vi "RT MainSam.vi"   [LabVIEW 2014]
uses:
  controls/UI DataSam.ctl
  <vilib>/RTwatchdog.llb/Watchdog expiration actions.ctl
  <vilib>/nisyscfg/nisyscfg.lvlib
types:
  T1 = typedef "UI DataSam.ctl" = cluster{"Message":string, "Data":variant}
  T2 = typedef "Watchdog expiration actions.ctl" = cluster{"reset":bool, "occurrence":bool, "trigger protocol":enum16{"active high", "active low", "open collector"}, "trigger line":enum16{"none", "line 0", "line 1", "line 2", "line 3", "line 4", "line 5", "line 6", "line 7", "SMB line 0"}, "disable watchdog on VI exit":bool}
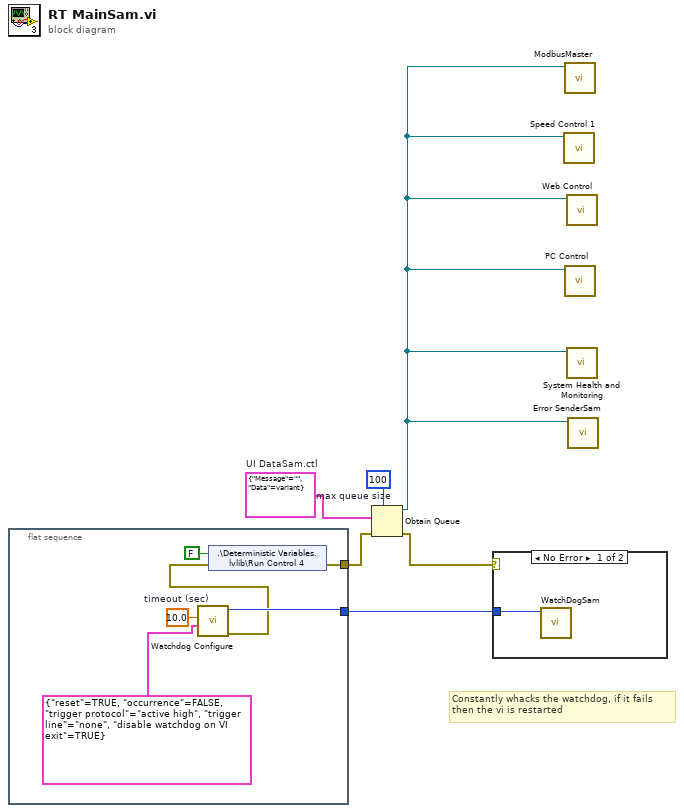
[diagram p0: block diagram]
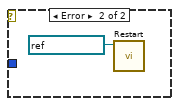
[diagram p2: hidden frame]
diagram:
  w5 = T1 {"Message"="", "Data"=variant}  # UI DataSam.ctl
  w6 = 100  # max queue size
  # "Constantly whacks the watchdog, if it fails\nthen the vi is restarted"
  n1 = flat-sequence {
    tunnel: [w12] -> w4
    tunnel: [w11] -> w2
    frame #0 {
      w9 = 10.0  # timeout (sec)
      n2 = call <vilib>:"Watchdog Configure.vi"("expiration actions"=T2 {"reset"=TRUE, "occurrence"=FALSE, "trigger protocol"=enum."active high", "trigger line"=enum."none", "disable watchdog on VI exit"=TRUE}, "timeout (1 sec)"=w9) -> ("error out"=w10:errorcluster, "watchdogID"=w11:u64)  [unwired: 2 in, 2 out]
      n3 = shared-variable ".\\Deterministic Variables.lvlib\\Run Control 4"(FALSE ("Run Control"), error in=w10) -> (error out=w12:errorcluster)
    }
  }
  n4 = Obtain Queue(max queue size (-1, unlimited)=w6, element data type=w5, error in (no error)=w4) -> (queue out=w1:refnum<queue>, error out=w3:errorcluster)  [unwired: 2 in, 1 out]
  n5 = case shown="No Error" w3 {
    tunnel: w2 -> [w13 _]
    frame No Error {
      n6 = call "WatchDogSam.vi"("watchdogID"=w13) -> ()  [unwired: 11 in]
    }
    frame Error {
      n7 = call <vilib>:"Restart.vi"("Session in"=refnum<k21> "localhost") -> ()  [unwired: 8 in, 3 out]
    }
  }
  n8 = call "Speed Control 1.vi"("queue in"=w1) -> ()  [unwired: 11 in]
  n9 = call "ModbusMaster.vi"("queue in"=w1) -> ()  [unwired: 11 in]
  n10 = call "PC Control.vi"("Queue in"=w1) -> ()  [unwired: 11 in]
  n11 = call "Web Control.vi"("Queue in"=w1) -> ()  [unwired: 11 in]
  n12 = call "System Health and Monitoring.vi"("queue in"=w1) -> ()  [unwired: 11 in]
  n13 = call "Error SenderSam.vi"("queue in"=w1) -> ()  [unwired: 11 in]
